vi "Write File.vi"(8 "error in (no error)":errorcluster, 10 "Parameters":refnum<class "Parameter.lvclass">[](array[class]), 11 "Parameter Generic File in":refnum<class "Parameter Generic File.lvclass">) -> (0 "error out":errorcluster, 3 "Parameter Generic File out":refnum<class "Parameter Generic File.lvclass">)   [LabVIEW 2016, in "CD Parameter Manager API.lvlib" / "Parameter Generic File.lvclass"]
uses:
  Parameter Generic File.lvclass
  Parameter Class/Parameter.lvclass
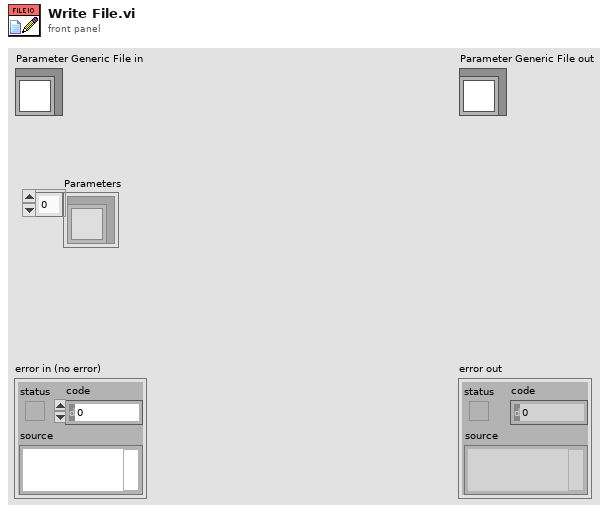
[diagram p1: front panel]
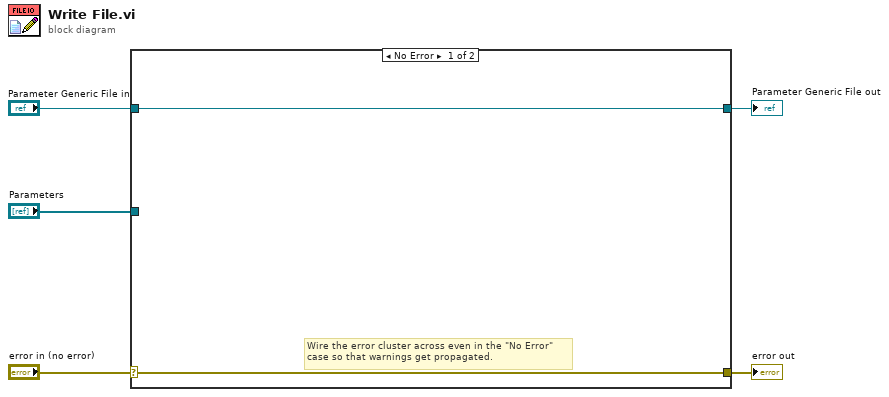
[diagram p0: block diagram]
diagram:
  n1 = case shown="No Error" "error in (no error)" {
    selector: "error in (no error)" -> [w7 w9]
    tunnel: [w7 w9] -> w4
    tunnel: [w6 w8] -> w2
    tunnel: "Parameter Generic File in" -> [w6 w8]
    tunnel: "Parameters" -> [_ _]
    frame No Error {
      # "Wire the error cluster across even in the \"No Error\"\ncase so that warnings get propagated."
    }
    frame Error {
    }
  }
  "error out" <- w4
  "Parameter Generic File out" <- w2
